vi "niSwitch Initialize with Topology for gRPC Session.vi"(5 "gRPC options":T2={"session name"="", "address (localhost)"="localhost", "port (31763)"=31763}, 7 "simulate (F)":bool, 8 "error in":errorcluster, 9 "reset device (T)":bool=TRUE, 10 "topology name":T1="Configured Topology", 11 "resource name":string) -> (0 "error out":errorcluster, 3 "session factory out":refnum<class "Session Factory.lvclass">)   [LabVIEW 2021, in "Session Management niSwitch.lvlib" / "Session Factory.lvclass"]
doc: "Initializes a new NI-Switch session on the specified NI gRPC Device Server and attaches to it. Returns a session factory object to be used in all subsequent NI-Switch calls."
uses:
  Session Factory.lvclass
  niSwitch gRPC Device Server.ctl
  <instrlib>/niSwitch/niSwitch.llb/niSwitch Topologies.ctl
  NI Switch Client/RPC Messages/niswitch_grpc_InitWithTopologyRequest.ctl
  NI Switch Client/RPC Messages/nidevice_grpc_SessionInitializationBehavior.ctl
  Session Factory.lvclass/Session Factory.ctl
  NI Switch Client/NI Switch Client.lvlib
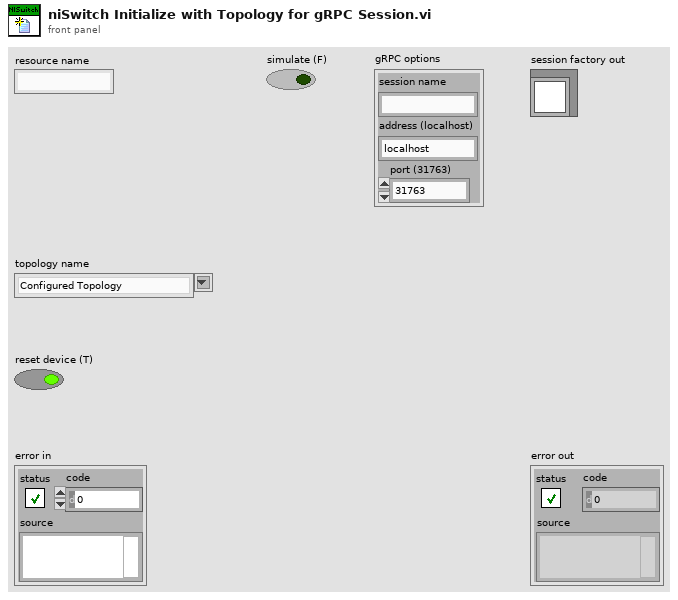
[diagram p1: front panel]
types:
  T1 = typedef "niSwitch Topologies.ctl" = string
  T2 = typedef "Session Management niSwitch.lvlib/Session Factory.lvclass/niSwitch gRPC Device Server.ctl" = cluster{"session name":string, "address (localhost)":string, "port (31763)":u32}
  T3 = typedef "NI Switch Client.lvlib/nidevice_grpc_SessionInitializationBehavior.ctl" = enum32{"SESSION_INITIALIZATION_BEHAVIOR_UNSPECIFIED", "SESSION_INITIALIZATION_BEHAVIOR_INITIALIZE_NEW", "SESSION_INITIALIZATION_BEHAVIOR_ATTACH_TO_EXISTING"}
  T4 = typedef "NI Switch Client.lvlib/niswitch_grpc_InitWithTopologyRequest.ctl" = cluster{"session_name":string, "resource_name":string, "topology":string, "simulate":bool, "reset_device":bool, "initialization_behavior":T3}
  T5 = typedef "grpc-lvsupport-release.lvlib/grpcId.ctl" = u64
  T6 = typedef "NI Switch Client.lvlib/niswitch_grpc_InitWithTopologyResponse.ctl" = cluster{"status":i32, "vi":T7, "error_message":string, "new_session_initialized":bool}
  T7 = typedef "NI Switch Client.lvlib/nidevice_grpc_Session.ctl" = cluster{"nidevice_grpc_Session_session":refnum<class "nidevice_grpc_Session_session.lvclass">}
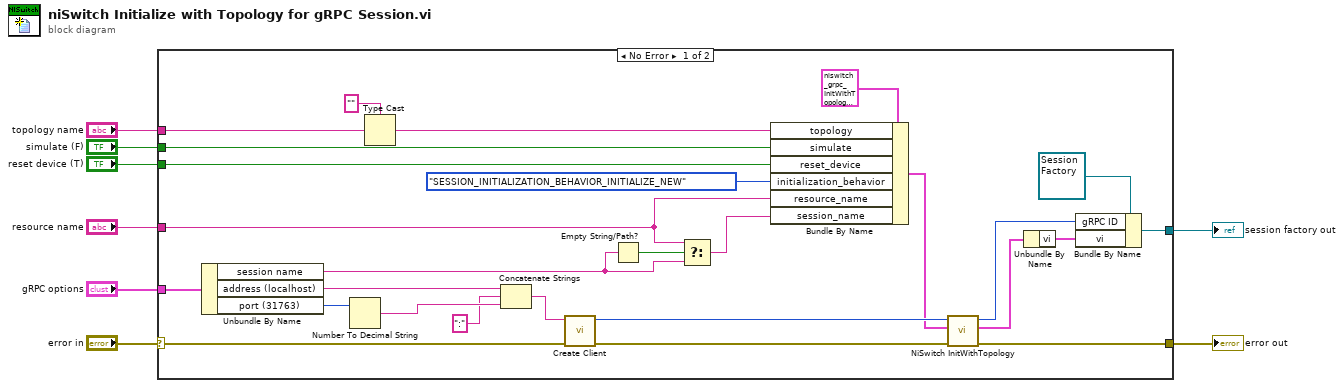
[diagram p0: block diagram]
diagram:
  n1 = case shown="No Error" "error in" {
    selector: "error in" -> [w31 w36]
    tunnel: [w28 w36] -> w8
    tunnel: "gRPC options" -> [w25 _]
    tunnel: "topology name" -> [w10 _]
    tunnel: "simulate (F)" -> [w21 _]
    tunnel: "reset device (T)" -> [w20 _]
    tunnel: "resource name" -> [w12 _]
    tunnel: [w9 _] -> w1
    frame No Error {
      n2 = Unbundle By Name(w25) -> ("session name"=w15:string, "address (localhost)"=w24:string, "port (31763)"=w23:u32)
      n3 = Number To Decimal String(number=w23) -> (decimal integer string=w30:string)  [unwired: 1 in]
      n4 = Type Cast(type="", x=w10) -> (*(type *) &x=w19:string)
      n5 = Concatenate Strings(w24, ":" ("string"), w30) -> (w26:string)
      n6 = call "Create Client.vi"("error in"=w31, "address"=w26) -> ("error out"=w29:errorcluster, "gRPC ID Out"=w35:T5)  [unwired: 8 in]
      n7 = Empty String/Path?(string/path=w15) -> (empty?=w14:bool)
      n8 = Select(t=w12, s=w14, f=w15) -> (s? t:f=w13:string)
      n9 = Bundle By Name(cluster=T4 {"session_name"="", "resource_name"="", "topology"="", "simulate"=FALSE, "reset_device"=FALSE, "initialization_behavior"=enum."SESSION_INITIALIZATION_BEHAVIOR_UNSPECIFIED"} ("Request Data"), "topology"=w19, "simulate"=w21, "reset_device"=w20, "initialization_behavior"=nidevice_grpc_SessionInitializationBehavior."SESSION_INITIALIZATION_BEHAVIOR_INITIALIZE_NEW", "resource_name"=w12, "session_name"=w13) -> (w22:T4)
      n10 = call "NiSwitch InitWithTopology.vi"("error in"=w29, "Request Data"=w22, "gRPC ID"=w35) -> ("error out"=w28:errorcluster, "Response Data"=w32:T6, "gRPC ID out"=w34:T5)  [unwired: 6 in]
      n11 = Unbundle By Name(w32) -> ("vi"=w33:T7)
      n12 = Bundle By Name(cluster=refnum<class "Session Factory.lvclass"> refnum ("Session Management niSwitch.lvlib:Session Factory.lvclass"), "gRPC ID"=w34, "vi"=w33) -> (w9:refnum<class "Session Factory.lvclass">)
    }
    frame Error {
    }
  }
  "error out" <- w8
  "session factory out" <- w1
